vi "23.Evd.8_Ask.4.vi"() -> ()   [LabVIEW 2025]
uses:
  <vilib>/Utility/file.llb/Write Delimited Spreadsheet (I64).vi
panel:
  in  "stop":bool
  out "Final state to be saved":dbl[](array[numeric])
  out "Live Engine Status":dbl[](array[numeric])
  in  "Engine 3":bool
  in  "Engine 2":bool
  in  "Engine 1":bool
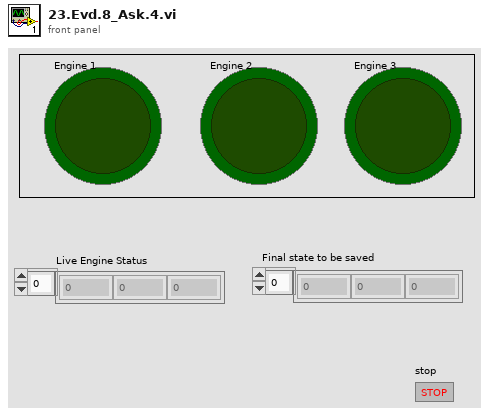
[diagram p1: front panel]
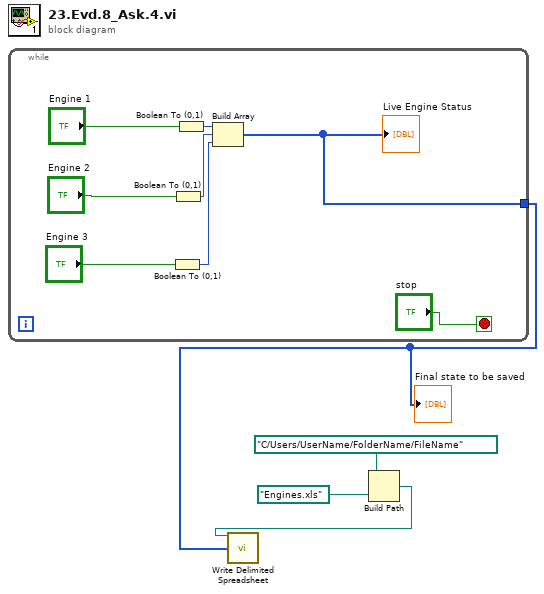
[diagram p0: block diagram]
diagram:
  n1 = while {
    tunnel: [w5] -> w4
    stop <- "stop" stop-if-true
    n2 = Boolean To (0,1)(Boolean="Engine 3") -> (0, 1=w7:i16)
    n3 = Boolean To (0,1)(Boolean="Engine 2") -> (0, 1=w9:i16)
    n4 = Boolean To (0,1)(Boolean="Engine 1") -> (0, 1=w11:i16)
    n5 = Build Array(w11, w9, w7) -> (w5:i16[])
    "Live Engine Status" <- w5
  }
  "Final state to be saved" <- w4
  n6 = Build Path(base path=path "C:/Users/UserName/FolderName/FileName" ("file path (dialog if empty)"), name or relative path=path "Engines.xls") -> (appended path=w1:path)
  n7 = call-poly <vilib>:"Write Delimited Spreadsheet.vi"("file path (dialog if empty)"=w1, "1D data"=w4) -> ()  [unwired: 12 in, 2 out]
